vi "Mode of Operation Value Change.vi"(8 "error in (no error)":errorcluster, 10 "Mode of Operation":T1, 11 "Doors Opening in":refnum<class "Doors Opening.lvclass">) -> (0 "error out":errorcluster, 3 "Doors Opening out":refnum<class "Doors Opening.lvclass">)   [LabVIEW 2020, in "Door Controller.lvlib" / "Doors Opening.lvclass"]
uses:
  Doors Opening.lvclass
  Door Interlocks/Mode of Operation.ctl
  Door Controller/Door Controller.lvclass
  Door Interlocks/Door Interlocks.lvclass
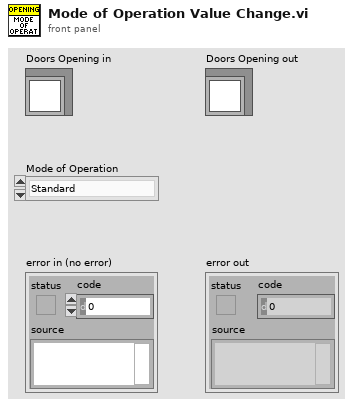
[diagram p1: front panel]
types:
  T1 = typedef "Door Interlocks.lvclass/Mode of Operation.ctl" = enum16{"Standard", "Interlock Override"}
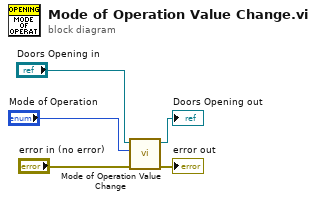
[diagram p0: block diagram]
diagram:
  n1 = call-parent "Mode of Operation Value Change.vi"("error in (no error)"="error in (no error)", "Mode of Operation"="Mode of Operation", "Door Controller in"="Doors Opening in") -> ("error out"=→"error out":errorcluster, "Door Controller out"=→"Doors Opening out":refnum<class "Doors Opening.lvclass">)  [unwired: 7 in]
